vi "匹配CH340串口.vi"() -> (3 "find list":string[](array[string]))   [LabVIEW 2016, in "DGUS.lvlib" / "DGUS.lvclass"]
uses:
  DGUS.lvclass
  <vilib>/Instr/_visa.llb/VISA Find Search Mode.ctl
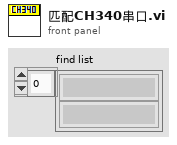
[diagram p1: front panel]
types:
  T1 = typedef "VISA Find Search Mode.ctl" = u32
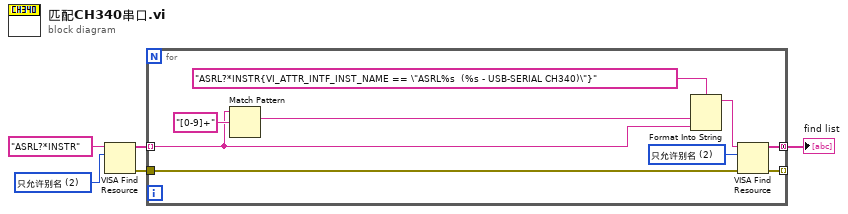
[diagram p0: block diagram]
diagram:
  w4 = T1 2 items=["仅允许规范名称"=0, "只允许别名"=2, "包含匹配别名"=3, "包含所有别名"=4] ("Search Mode")
  n1 = VISA Find Resource(10:w4, 11:"ASRL?*INSTR" ("表达式(\"?*\")")) -> (0:w1:errorcluster, 3:w3:string[])  [unwired: 1 in, 1 out]
  n2 = for {
    tunnel: w3 -> [w11] mode=indexing
    tunnel: [w8] -> w2 mode=concatenating
    tunnel: [w7] -> _ mode=indexing
    tunnel: w1 -> [w6]
    w9 = T1 2 items=["仅允许规范名称"=0, "只允许别名"=2, "包含匹配别名"=3, "包含所有别名"=4] ("Search Mode")
    n3 = Match Pattern(string=w11, regular expression="[0-9]+" ("正则表达式")) -> (match substring=w12:string)  [unwired: 1 in, 3 out]
    n4 = Format Into String(format string="ASRL?*INSTR{VI_ATTR_INTF_INST_NAME == \"ASRL%s  (%s - USB-SERIAL CH340)\"}" ("表达式(\"?*\")"), w12, w11) -> (resulting string=w10:string)  [unwired: 2 in, 1 out]
    n5 = VISA Find Resource(8:w6, 10:w9, 11:w10) -> (0:w7:errorcluster, 3:w8:string[])  [unwired: 1 out]
  }
  "find list" <- w2
